vi "Get VS item parameter map.vi"(8 "error in (no error)":errorcluster, 11 "Iten refs in":T4=18446744073709551615 format="%.0x") -> (0 "error out":errorcluster, 1 "Found?":bool, 2 "param config out":T1[](array[typedef]), 3 "Iten refs out":T4=18446744073709551615 format="%.0x")   [LabVIEW 2020, in "Ballard 1553 System Explorer.lvlib"]
uses:
  <vilib>/NI VeriStand/Custom Device API/Custom Device Item Ref.ctl
  Shared/EncodeDecode/_typedefs/parameter_config_type.ctl
  Shared/EncodeDecode/_typedefs/parameter_config_type_type.ctl
  Shared/EncodeDecode/_typedefs/parameter_config_encoding_type.ctl
  Shared/Controls and Global/Global.vi
  <vilib>/NI VeriStand/Custom Device API/Get Item Property (Variant).vi
  Ballard 1553 System Explorer.lvlib
  Shared/Ballard 1553 Shared.lvlib
  <vilib>/NI VeriStand/Custom Device API/Custom Device API.lvlib
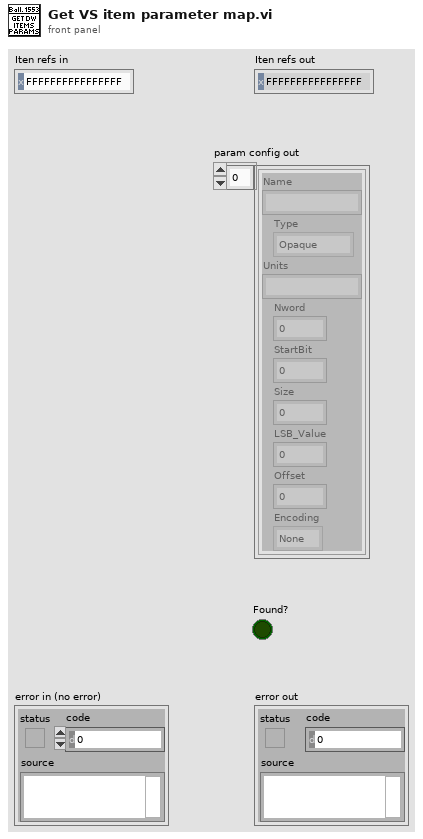
[diagram p1: front panel]
types:
  T1 = typedef "parameter_config_type.ctl" = cluster{"Name":string, "Type":T2, "Units":string, "Nword":i32, "StartBit":i32, "Size":i32, "LSB_Value":i32, "Offset":i32, "Encoding":T3}
  T2 = typedef "parameter_config_type_type.ctl" = enum16{"Opaque", "Enum", "Float", "Integer", "Bcd", "Bool"}
  T3 = typedef "parameter_config_encoding_type.ctl" = enum16{"None", "2-complement", "Unsigned"}
  T4 = typedef "Custom Device API.lvlib/Custom Device Item Ref.ctl" = u64
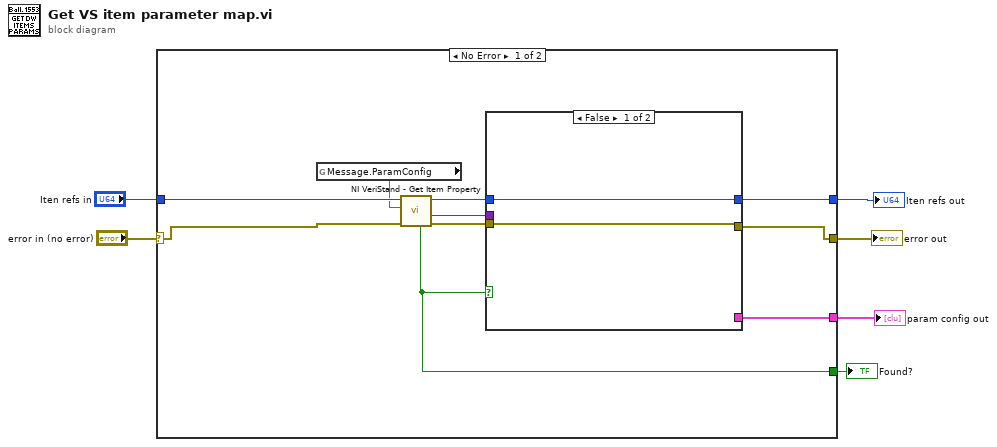
[diagram p0: block diagram]
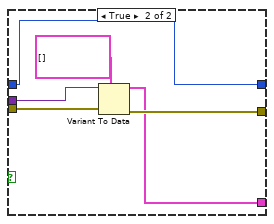
[diagram p2: hidden frame]
diagram:
  n1 = case shown="No Error" "error in (no error)" {
    selector: "error in (no error)" -> [w15 w26]
    tunnel: [w13 w26] -> w5
    tunnel: [w14 w25] -> w4
    tunnel: "Iten refs in" -> [w16 w25]
    tunnel: [w8 _] -> w1
    tunnel: [w7 _] -> w2
    frame No Error {
      n2 = global read "Global.vi" "Message.ParamConfig"() -> (w12:string)
      n3 = call-poly <vilib>:"NI VeriStand - Get Item Property.vi"("error in (no error)"=w15, "Property Name"=w12, "Item Ref in"=w16) -> ("error out"=w10:errorcluster, "Value"=w9:variant, "Item Ref out"=w11:T4, "Found?"=w7:bool)  [unwired: 5 in]
      n4 = case shown="False" w7 {
        tunnel: w11 -> [w18 w21]
        tunnel: w10 -> [w17 w23]
        tunnel: w9 -> [_ w24]
        tunnel: [w18 w21] -> w14
        tunnel: [w17 w20] -> w13
        tunnel: [_ w19] -> w8
        frame False {
        }
        frame True {
          n5 = Variant To Data(error in=w23, type=T1[] [] ("Array"), Variant=w24) -> (data=w19:T1[], error out=w20:errorcluster)
        }
      }
    }
    frame Error {
    }
  }
  "error out" <- w5
  "Iten refs out" <- w4
  "param config out" <- w1
  "Found?" <- w2
